vi "file list -- accumulate V4.vi"(11 "file path":path=path "/snowfall/Users/arcadi/Desktop/Ultrasound/Experiment/YBCO_4/Round1/Sweep12/June_2011/062511/221.16400K_300_3100_001_062511.dat") -> (0 "timestamp":dbl[](array[numeric]), 2 "sweep file name array":T1[](array[typedef]), 3 "temperatures":dbl[](array[numeric]))   [LabVIEW 2012]
uses:
  sweep file name.ctl
panel:
  in  "dummy 2":T1={"temperature"=0.0, "temperature str"="", "file path"=path "/snowfall/Users/arcadi/Desktop/Ultrasound/Experiment/YBCO_4/Round1/Sweep12/June_2011/062511/221.16400K_300_3100_001_062511.dat", "last mod"=timestamp(0 s since 1904-01-01), "file name str"="", "mod time(min)"=0.0, "file format"=enum.""}
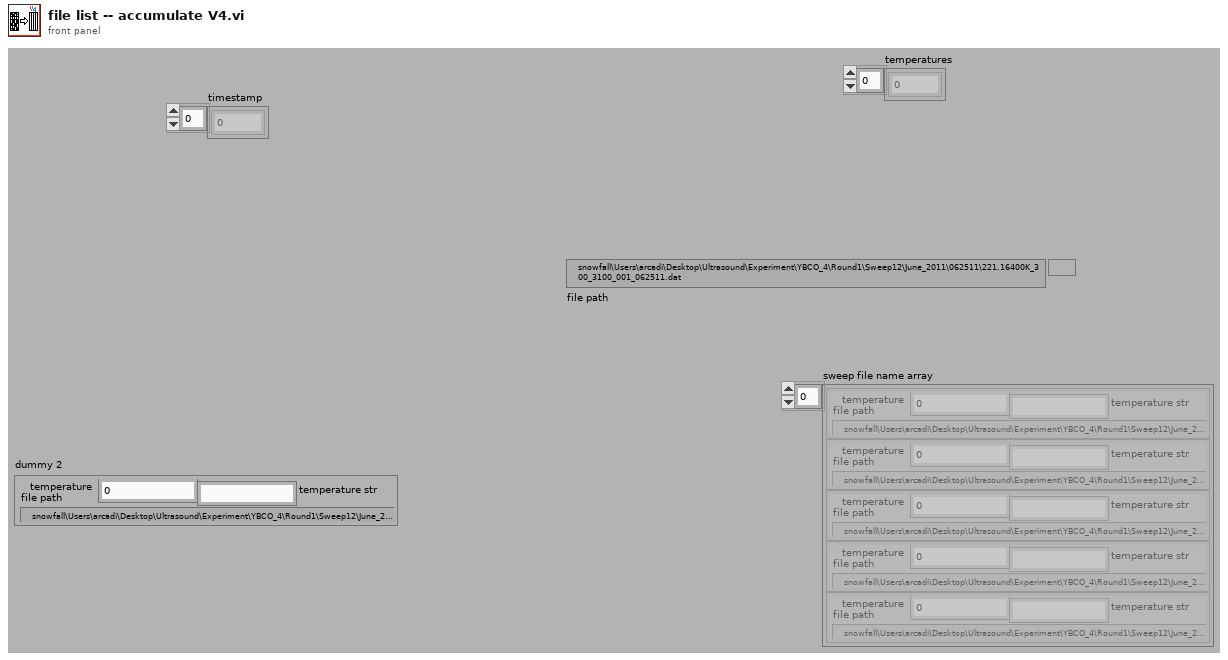
[diagram p1: front panel]
types:
  T1 = typedef "sweep file name.ctl" = cluster{"temperature":dbl, "temperature str":string, "file path":path, "last mod":timestamp, "file name str":string, "mod time(min)":dbl, "file format":enum16{"", "ascii", "binary"}}
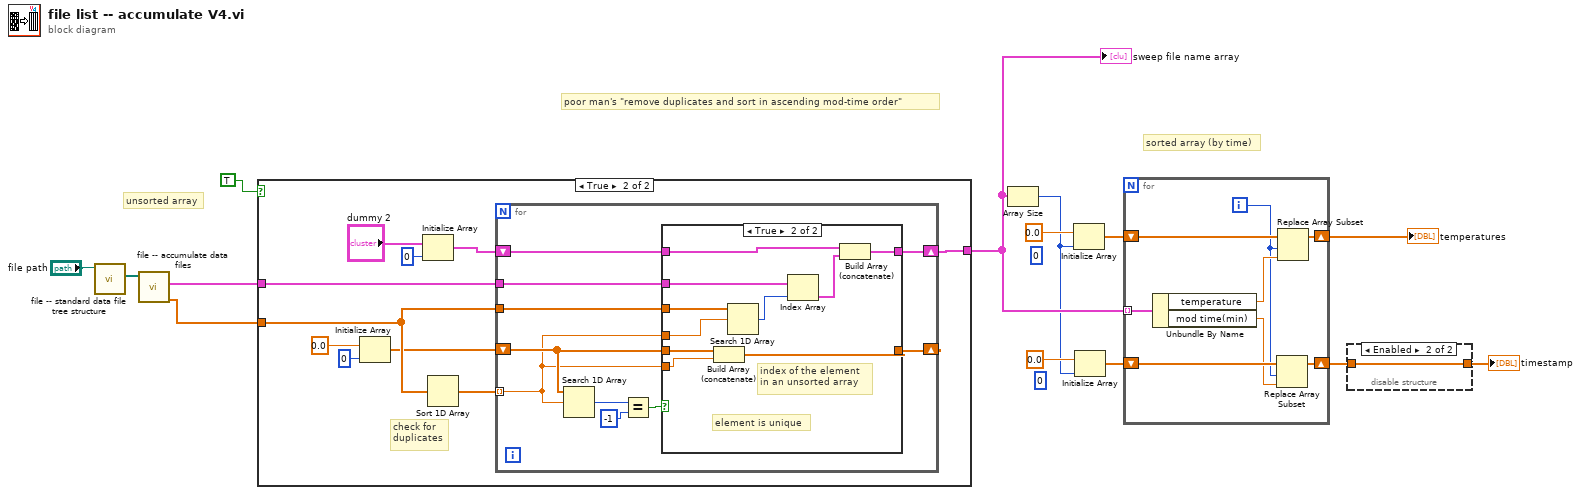
[diagram p0: block diagram]
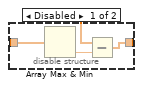
[diagram p2: hidden frame]
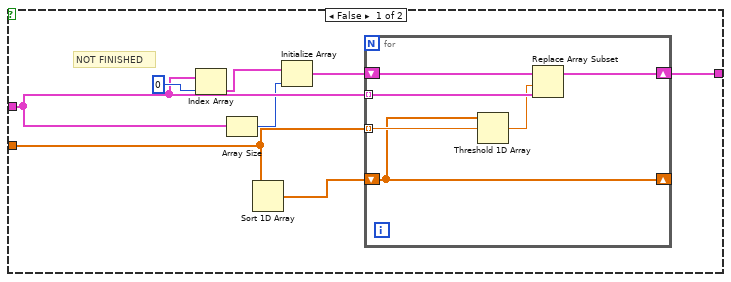
[diagram p3: hidden frame]
diagram:
  (unwired) 0 ("dimension size")
  (unwired) 0 ("dimension size")
  # "sorted array (by time)"
  # "unsorted array"
  # "poor man's \"remove duplicates and sort in ascending mod-time order\""
  n1 = call "file -- standard data file tree structure.vi"("folder path"="file path") -> ("Array"=w3:path[])  [unwired: 10 in]
  n2 = call "file -- accumulate data files.vi"("list of <mmddyy> folders"=w3) -> ("timestamp array"=w4:dbl[], "sweep file name  array"=w5:T1[])  [unwired: 9 in]
  n3 = case shown="True" TRUE {
    tunnel: w4 -> [w21 w32]
    tunnel: w5 -> [w18 w37]
    tunnel: [w15 w36] -> w2
    frame False {
      # "NOT FINISHED"
      n4 = Index Array(array=w18, index=0) -> (element=w19:T1)
      n5 = Array Size(array=w18) -> (size(s)=w17:i32)
      n6 = Sort 1D Array(array=w21) -> (sorted array=w22:dbl[])
      n7 = Initialize Array(w19, w17) -> (w16:T1[])
      n8 = for {
        tunnel: w18 -> [w25] mode=indexing
        tunnel: w21 -> [w28] mode=indexing
        shift-right: [w27] -> _
        shift-left: w22 -> [w27]
        shift-right: [w23] -> w15
        shift-left: w16 -> [w26]
        n9 = Threshold 1D Array(2:w28, 3:w27) -> (0:w24:dbl)  [unwired: 1 in]
        n10 = Replace Array Subset(array=w26, new element=w25, index=w24) -> (w23:T1[])
      }
    }
    frame True {
      # "check for \nduplicates"
      n11 = Initialize Array(0.0 ("dimension size"), 0 ("dimension size")) -> (w29:dbl[])
      n12 = Initialize Array("dummy 2", 0 ("dimension size")) -> (w33:T1[])
      n13 = Sort 1D Array(array=w32) -> (sorted array=w38:dbl[])
      n14 = for {
        shift-right: [w45] -> w36
        shift-left: w33 -> [w44]
        shift-right: [w43] -> _
        shift-left: w29 -> [w42]
        tunnel: w38 -> [w39] mode=indexing
        tunnel: w32 -> [w41]
        tunnel: w37 -> [w40]
        n15 = Search 1D Array(1D array=w42, element=w39) -> (index of element=w48:i32)  [unwired: 1 in]
        n16 = Equal?(x=w48, y=-1) -> (x = y?=w46:bool)
        n17 = case shown="True" w46 {
          tunnel: [w50 w59] -> w45
          tunnel: w44 -> [w50 w60]
          tunnel: [w49 w51] -> w43
          tunnel: w42 -> [w49 w53]
          tunnel: w41 -> [_ w58]
          tunnel: w39 -> [_ w57]
          tunnel: w40 -> [_ w55]
          tunnel: w39 -> [_ w52]
          frame False {
            # "element is not unique"
          }
          frame True {
            # "index of the element \nin an unsorted array"
            # "element is unique"
            n18 = Build Array (concatenate)(w53, w52) -> (w51:dbl[])
            n19 = Search 1D Array(1D array=w58, element=w57) -> (index of element=w56:i32)  [unwired: 1 in]
            n20 = Index Array(array=w55, index=w56) -> (element=w54:T1)
            n21 = Build Array (concatenate)(w60, w54) -> (w59:T1[])
          }
        }
      }
    }
  }
  "sweep file name array" <- w2
  n22 = Array Size(array=w2) -> (size(s)=w1:i32)
  n23 = Initialize Array(0.0 ("dimension size"), w1) -> (w12:dbl[])
  n24 = Initialize Array(0.0 ("dimension size"), w1) -> (w10:dbl[])
  n25 = for {
    tunnel: w2 -> [w68] mode=indexing
    shift-right: [w64] -> w9
    shift-left: w12 -> [w67]
    shift-right: [w65] -> w8
    shift-left: w10 -> [w66]
    i -> [w61]
    n26 = Unbundle By Name(w68) -> ("temperature"=w63:dbl, "mod time(min)"=w62:dbl)
    n27 = Replace Array Subset(array=w66, new element=w62, index=w61) -> (w65:dbl[])
    n28 = Replace Array Subset(array=w67, new element=w63, index=w61) -> (w64:dbl[])
  }
  "temperatures" <- w9
  n29 = disable-structure shown="Enabled" {
    disable-tunnel: w8 -> [w70 w72]
    disable-tunnel: [w69 w72] -> w7
    frame Disabled {
      n30 = Array Max & Min(array=w70) -> (min value=w71:dbl)  [unwired: 3 out]
      n31 = Subtract(x=w70, y=w71) -> (x-y=w69:dbl[])
    }
    frame Enabled {
    }
  }
  "timestamp" <- w7
